vi "Untitled 7.vi"() -> ()   [LabVIEW 2014]
panel:
  out "NaN/Path/Refnum?":bool
  out "error out":errorcluster
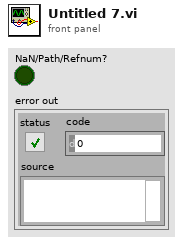
[diagram p1: front panel]
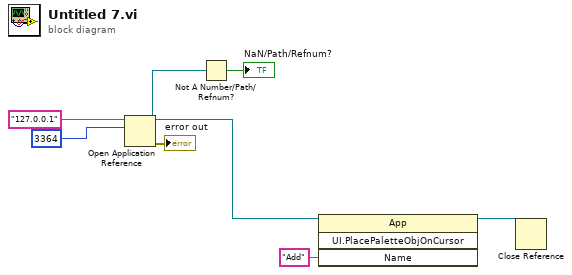
[diagram p0: block diagram]
diagram:
  n1 = Open Application Reference(10:u16 3364 ("port number or service name (3363)"), 11:"127.0.0.1" ("machine name (\"\":  open local reference)")) -> (0:→"error out":errorcluster, 3:w3:refnum<vi>)  [unwired: 2 in]
  n2 = Not A Number/Path/Refnum?(number/path/refnum=w3) -> (NaN/Path/Refnum?=→"NaN/Path/Refnum?":bool)
  n3 = invoke class="App" method="UI.PlacePaletteObjOnCursor"(reference=w3, "Name"="Add" ("Ctl or Function Name")) -> (reference out=w2:refnum<vi>)  [unwired: 2 in, 3 out]
  n4 = Close Reference(reference=w2) -> ()  [unwired: 1 in, 1 out]
